vi "Move Downfield.vi"(6 "toGear":dbl, 8 "error in (no error)":errorcluster, 9 "gearDistance":dbl, 10 "Position":string, 11 "PID gains":T1) -> (0 "error out":errorcluster)   [LabVIEW 2016]
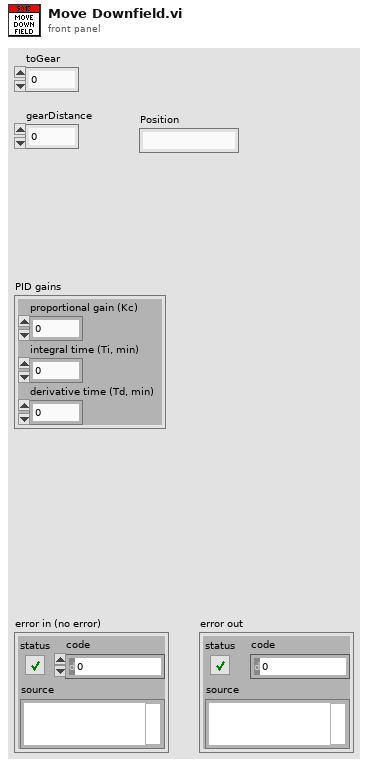
[diagram p1: front panel]
types:
  T1 = cluster{"proportional gain (Kc)":dbl, "integral time (Ti, min)":dbl, "derivative time (Td, min)":dbl}
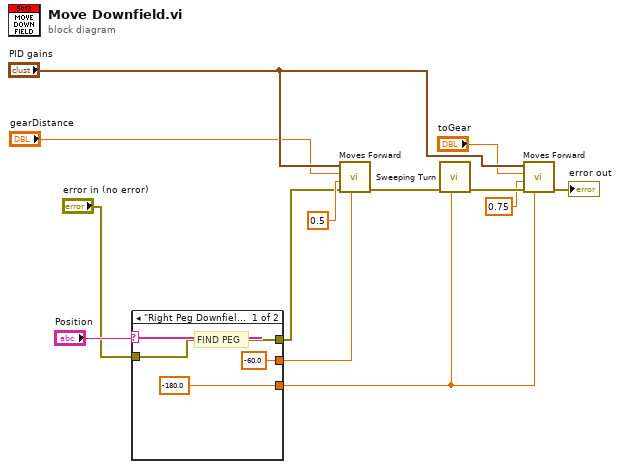
[diagram p0: block diagram]
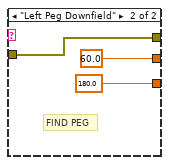
[diagram p2: hidden frame]
diagram:
  n1 = case shown="\"Right Peg Downfield\", Default" "Position" {
    tunnel: "error in (no error)" -> [w15 w18]
    tunnel: [w15 w18] -> w4
    tunnel: [-180.0 ("upper limit right") 180.0 ("upper limit left")] -> w1
    tunnel: [-60.0 ("upper limit left") 60.0 ("upper limit left")] -> w2
    frame "Right Peg Downfield", Default {
      # "FIND PEG"
    }
    frame "Left Peg Downfield" {
      # "FIND PEG"
    }
  }
  n2 = call "Moves Forward.vi"("yaw setpoint"=w2, "error in (no error)"=w4, "Speed"=0.5, "forwardDistance"="gearDistance", "PID gains"="PID gains") -> ("error out"=w3:errorcluster)  [unwired: 4 in, 2 out]
  n3 = call "Sweeping Turn.vi"("upper angle limit"=w1, "error in"=w3) -> ("error out"=w11:errorcluster)  [unwired: 9 in]
  n4 = call "Moves Forward.vi"("yaw setpoint"=w1, "error in (no error)"=w11, "Speed"=0.75, "forwardDistance"="toGear", "PID gains"="PID gains") -> ("error out"=→"error out":errorcluster)  [unwired: 4 in, 2 out]
